vi "AFG3352XGUI.constructor.vi"(0 "name":string, 2 "data in":string, 5 "error in (no error)":errorcluster) -> (14 "i ref out":refnum<vi>, 16 "data out":string, 19 "error out":errorcluster)   [LabVIEW 2014, in "AFG3352XGUI.lvlib"]
doc: "constructor of the AFGBaseGUI class"
uses:
  AFG3352XGUI.lvlib
  CS_Core/CSSystem/CSSystemLib/CSSystemLib.lvlib
  CS_Core/GUIs/GOGUserGUIs/DeviceBaseGUI/DeviceBaseGUI.lvlib
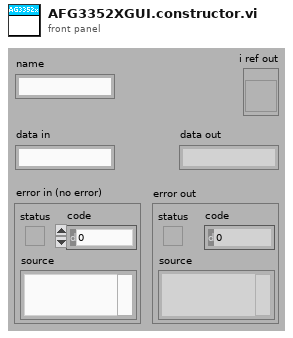
[diagram p1: front panel]
types:
  T1 = enum16{"SetAttribute", "GetAttribute", "CreateAttribute", "DestroyAttribute", "DestroyAllAtributes"}
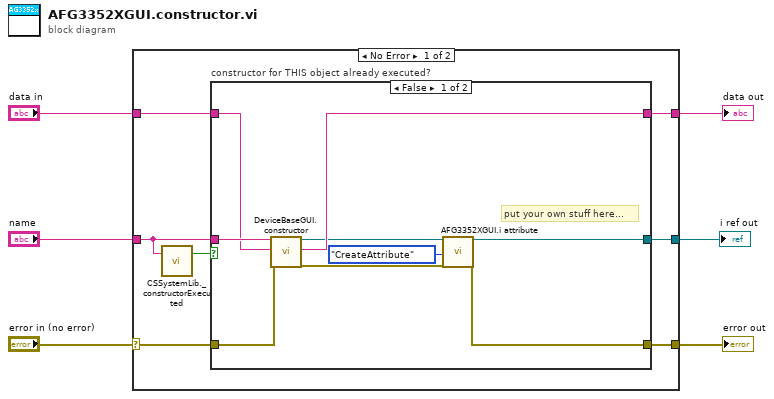
[diagram p0: block diagram]
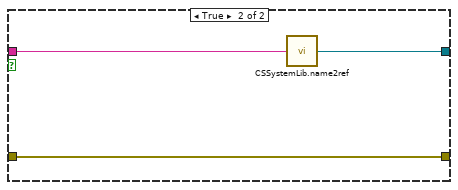
[diagram p2: hidden frame]
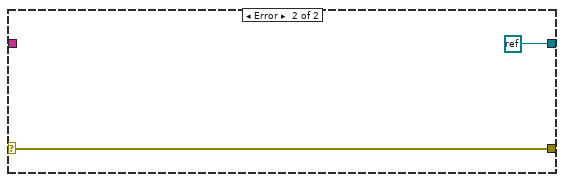
[diagram p3: hidden frame]
diagram:
  n1 = case shown="No Error" "error in (no error)" {
    selector: "error in (no error)" -> [w10 w26]
    tunnel: "data in" -> [w13 _]
    tunnel: "name" -> [w9 _]
    tunnel: [w12 refnum<k0> refnum ("Not a Refnum Constant")] -> w4
    tunnel: [w11 w26] -> w3
    tunnel: [w7 _] -> w1
    frame No Error {
      n2 = call "CSSystemLib._constructorExecuted.vi"("name"=w9) -> ("constructor executed?"=w8:bool)  [unwired: 18 in]
      n3 = case "constructor for THIS object already executed?" shown="False" w8 {
        tunnel: w13 -> [w20 _]
        tunnel: w9 -> [w21 w25]
        tunnel: [w19 w24] -> w12
        tunnel: [w14 w23] -> w11
        tunnel: w10 -> [w16 w23]
        tunnel: [w18 _] -> w7
        frame False {
          # "put your own stuff here..."
          n4 = call "DeviceBaseGUI.constructor.vi"("name"=w21, "data in"=w20, "error in (no error)"=w16) -> ("i ref out"=w17:refnum<vi>, "data out"=w18:string, "error out"=w15:errorcluster)  [unwired: 14 in]
          n5 = call "AFG3352XGUI.i attribute.vi"("VI Refnum"=w17, "Action"=T1."CreateAttribute", "error in (no error)"=w15) -> ("VI Refnum out"=w19:refnum<vi>, "error out"=w14:errorcluster)  [unwired: 14 in, 1 out]
        }
        frame True {
          n6 = call "CSSystemLib.name2ref.vi"("name"=w25) -> ("obj refnum"=w24:refnum<vi>)
        }
      }
    }
    frame Error {
    }
  }
  "i ref out" <- w4
  "error out" <- w3
  "data out" <- w1
